vi "Delet Tests.vi"() -> ()   [LabVIEW 2020]
uses:
  FGV Map/Controls/FGV Map Core State.ctl
  FGV Map.lvlib
panel:
  out "Instance Out 3":map{string, variant}(c390)
  out "Deleted Instance":map{string, variant}(c390)
  out "Instance Out 2":map{string, variant}(c390)
  out "Deleted Data":variant
  out "Instance Out":map{string, variant}(c390)
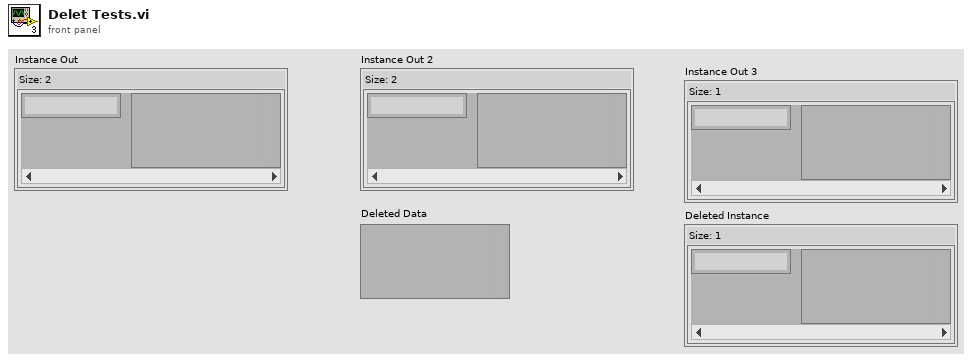
[diagram p1: front panel]
types:
  T1 = typedef "FGV Map.lvlib/FGV Map Core State.ctl" = enum16{"Init", "Set Instance (Unlock)", "Get Instance", "Get Instance (Lock)", "Unlock", "Get All Instances", "Delete Instance"}
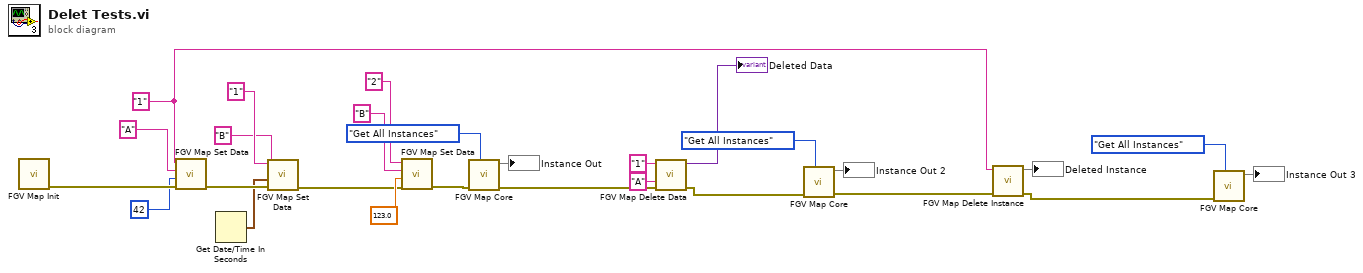
[diagram p0: block diagram]
diagram:
  w5 = "1" ("Instance Key")
  n1 = call "FGV Map Init.vi"() -> ("error out"=w27:errorcluster)  [unwired: 11 in]
  n2 = call "FGV Map Set Data.vi"("error in (no error)"=w27, "Data In"=42, "Data Key"="A", "Instance Key"=w5) -> ("error out"=w21:errorcluster)  [unwired: 5 in, 2 out]
  n3 = Get Date/Time In Seconds() -> (seconds since 1Jan1904=w17:timestamp)
  n4 = call "FGV Map Set Data.vi"("error in (no error)"=w21, "Data In"=w17, "Data Key"="B", "Instance Key"="1") -> ("error out"=w20:errorcluster)  [unwired: 5 in, 2 out]
  n5 = call "FGV Map Set Data.vi"("error in (no error)"=w20, "Data In"=123.0, "Data Key"="B", "Instance Key"="2") -> ("error out"=w16:errorcluster)  [unwired: 5 in, 2 out]
  n6 = call "FGV Map Core.vi"("FGV State"=FGV_Map_Core_State."Get All Instances", "error in"=w16) -> ("error out"=w13:errorcluster, "Instance Out"=→"Instance Out":map{string, variant})  [unwired: 5 in, 3 out]
  n7 = call "FGV Map Delete Data.vi"("error in (no error)"=w13, "Data Key"="A", "Instance Key"="1") -> ("error out"=w7:errorcluster, "Deleted Data"=→"Deleted Data":variant)  [unwired: 6 in, 1 out]
  n8 = call "FGV Map Core.vi"("FGV State"=FGV_Map_Core_State."Get All Instances", "error in"=w7) -> ("error out"=w6:errorcluster, "Instance Out"=→"Instance Out 2":map{string, variant})  [unwired: 5 in, 3 out]
  n9 = call "FGV Map Delete Instance.vi"("error in (no error)"=w6, "Instance Key"=w5) -> ("error out"=w1:errorcluster, "Deleted Instance"=→"Deleted Instance":map{string, variant})  [unwired: 7 in, 1 out]
  n10 = call "FGV Map Core.vi"("FGV State"=FGV_Map_Core_State."Get All Instances", "error in"=w1) -> ("Instance Out"=→"Instance Out 3":map{string, variant})  [unwired: 5 in, 4 out]
